vi "Bundle Wheel PID SetPoint Test.vi"(10 "array":dbl[](array[numeric])) -> (0 "element 4":dbl, 1 "element 2":dbl, 3 "element":dbl, 4 "element 5":dbl)   [LabVIEW 2015]
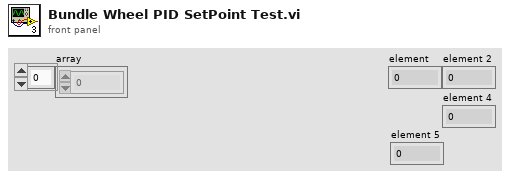
[diagram p1: front panel]
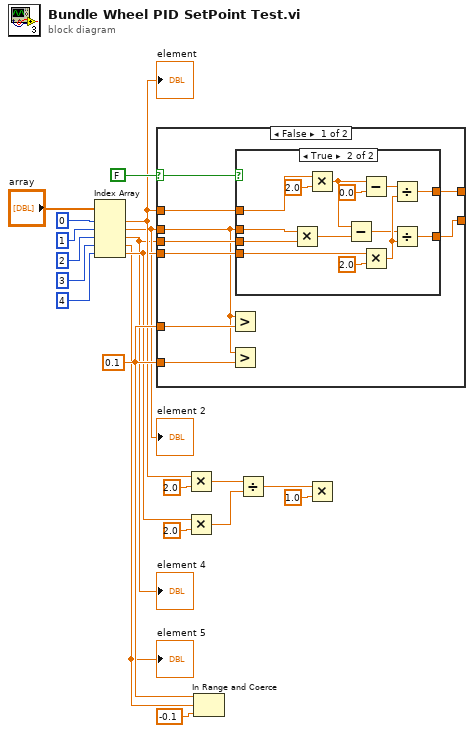
[diagram p0: block diagram]
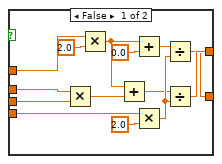
[diagram p2: hidden frame]
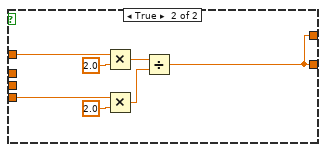
[diagram p3: hidden frame]
diagram:
  w13 = 0.1 ("upper limit")
  n1 = Index Array(array="array", index #1=0 ("index"), index #2=1 ("index"), index #3=2 ("index"), index #4=3 ("index"), index #5=4 ("index")) -> (element #1=w11:dbl, element #2=w8:dbl, element #3=w7:dbl, element #4=w6:dbl, element #5=w10:dbl)
  "element" <- w11
  "element 2" <- w8
  "element 4" <- w7
  "element 5" <- w6
  n2 = case shown="False" FALSE {
    selector: FALSE -> [w21 _]
    tunnel: w13 -> [w29 _]
    tunnel: [w28 w60] -> _
    tunnel: [w27 w60] -> _
    tunnel: w8 -> [w23 _]
    tunnel: w10 -> [w25 w59]
    tunnel: w7 -> [w24 _]
    tunnel: w11 -> [w26 w58]
    tunnel: w13 -> [w22 _]
    frame False {
      n3 = Greater?(x=w23, y=w29) -> ()  [unwired: 1 out]
      n4 = Greater?(x=w23, y=w22) -> ()  [unwired: 1 out]
      n5 = case shown="True" w21 {
        tunnel: [w37 w51] -> w28
        tunnel: [w36 w50] -> w27
        tunnel: w26 -> [w33 w47]
        tunnel: w25 -> [w30 w46]
        tunnel: w23 -> [w32 w45]
        tunnel: w24 -> [w31 w44]
        frame False {
          n6 = Multiply(x=w32, y=w31) -> (x*y=w35:dbl)
          n7 = Multiply(x=w33, y=2.0) -> (x*y=w40:dbl)
          n8 = Add(x=w40, y=w35) -> (x+y=w42:dbl)
          n9 = Add(x=w40, y=0.0) -> (x+y=w41:dbl)
          n10 = Multiply(x=w30, y=2.0) -> (x*y=w43:dbl)
          n11 = Divide(x=w41, y=w43) -> (x/y=w36:dbl)
          n12 = Divide(x=w42, y=w43) -> (x/y=w37:dbl)
        }
        frame True {
          n13 = Multiply(x=w45, y=w44) -> (x*y=w49:dbl)
          n14 = Multiply(x=w47, y=2.0) -> (x*y=w54:dbl)
          n15 = Subtract(x=w54, y=w49) -> (x-y=w55:dbl)
          n16 = Subtract(x=w54, y=0.0) -> (x-y=w56:dbl)
          n17 = Multiply(x=w46, y=2.0) -> (x*y=w57:dbl)
          n18 = Divide(x=w56, y=w57) -> (x/y=w51:dbl)
          n19 = Divide(x=w55, y=w57) -> (x/y=w50:dbl)
        }
      }
    }
    frame True {
      n20 = Multiply(x=w58, y=2.0) -> (x*y=w61:dbl)
      n21 = Multiply(x=w59, y=2.0) -> (x*y=w64:dbl)
      n22 = Divide(x=w61, y=w64) -> (x/y=w60:dbl)
    }
  }
  n23 = Multiply(x=w11, y=2.0) -> (x*y=w18:dbl)
  n24 = Multiply(x=w10, y=2.0) -> (x*y=w15:dbl)
  n25 = In Range and Coerce(upper limit=w13, x=w6, lower limit=-0.1) -> ()  [unwired: 2 out]
  n26 = Divide(x=w18, y=w15) -> (x/y=w14:dbl)
  n27 = Multiply(x=w14, y=1.0) -> ()  [unwired: 1 out]
